vi "TestAndSetNextTestCasePointer.vi"(0 "TestSeqClass in":refnum<class "TestSeqClass.lvclass">, 11 "error in (no error)":errorcluster) -> (4 "TestSeqClass out":refnum<class "TestSeqClass.lvclass">, 8 "Continue":bool, 10 "Pointer at end":bool, 15 "error out":errorcluster)   [LabVIEW 2019, in "TestSeqClass.lvclass"]
uses:
  TestSeqClass.lvclass
  Typedef/TestStatus.ctl
  TestSeqClass.lvclass/TestSeqClass.ctl
  TestMeasureStep/TestMeasureStep.lvclass
  Read CurrentTestPointer.vi
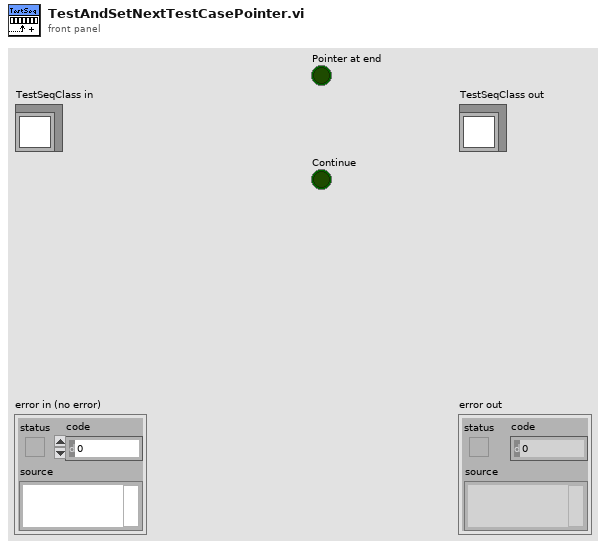
[diagram p1: front panel]
types:
  T1 = typedef "TestStatus.ctl" = enum16{"Not Executed", "Passed", "Failed", "Inconclusive", "Processing"}
  T2 = typedef "TestSeqType.ctl" = refnum<class "TestMeasureStep.lvclass">[]
  T3 = typedef "TestSeqClass.lvclass/TesstepType.ctl" = cluster{"TestName":string, "Meas":dbl, "Min ":dbl, "Max":dbl, "TestStatus":T1, "StringLimit":string, "StringMeas":string, "Unit":string}
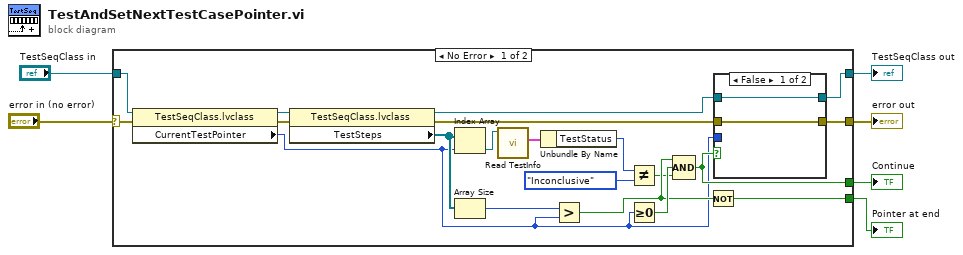
[diagram p0: block diagram]
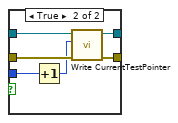
[diagram p2: hidden frame]
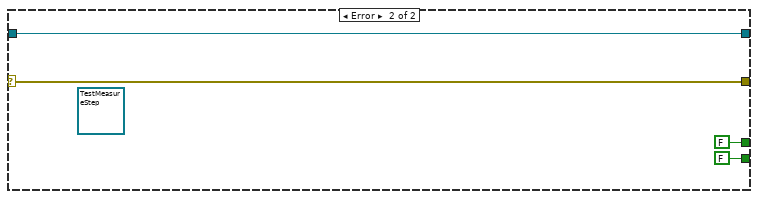
[diagram p3: hidden frame]
diagram:
  n1 = case shown="No Error" "error in (no error)" {
    selector: "error in (no error)" -> [w22 w38]
    tunnel: [w24 w38] -> w5
    tunnel: [w25 w37] -> w3
    tunnel: "TestSeqClass in" -> [w23 w37]
    tunnel: [w26 FALSE] -> w2
    tunnel: [w14 FALSE] -> w1
    frame No Error {
      n2 = property class="TestSeqClass.lvclass"(reference=w23, error in=w22) -> (reference out=w21:refnum<class "TestSeqClass.lvclass">, error out=w20:errorcluster, "CurrentTestPointer"=w12:u32)
      n3 = property class="TestSeqClass.lvclass"(reference=w21, error in=w20) -> (reference out=w17:refnum<class "TestSeqClass.lvclass">, error out=w16:errorcluster, "TestSteps"=w13:T2)
      n4 = Index Array(array=w13, index=w12) -> (element=w11:refnum<class "TestMeasureStep.lvclass">)
      n5 = Array Size(array=w13) -> (size(s)=w19:i32)
      n6 = call-dynamic "Read TestInfo.vi"("TestMeasureStep in"=w11) -> ("TestInfo 2"=w10:T3)  [unwired: 8 in, 2 out]
      n7 = Unbundle By Name(w10) -> ("TestStatus"=w9:T1)
      n8 = Greater?(x=w19, y=w12) -> (0:w15:bool)
      n9 = Not Equal?(x=w9, y=TestStatus."Inconclusive") -> (x != y?=w7:bool)
      n10 = Greater Or Equal To 0?(x=w12) -> (x >= 0?=w18:bool)
      n11 = Compound Arithmetic op=AND(w15, w18, w7) -> (w26:bool)
      n12 = Not(x=w15) -> (.not. x?=w14:bool)
      n13 = case shown="False" w26 {
        tunnel: w17 -> [w28 w34]
        tunnel: w16 -> [w27 w32]
        tunnel: w12 -> [_ w30]
        tunnel: [w28 w33] -> w25
        tunnel: [w27 w31] -> w24
        frame False {
        }
        frame True {
          n14 = Increment(x=w30) -> (x+1=w29:u32)
          n15 = call "Write CurrentTestPointer.vi"("error in (no error)"=w32, "CurrentTestPointer"=w29, "TestSeqClass in"=w34) -> ("error out"=w31:errorcluster, "TestSeqClass out"=w33:refnum<class "TestSeqClass.lvclass">)  [unwired: 7 in]
        }
      }
    }
    frame Error {
      (unwired) refnum<class "TestMeasureStep.lvclass"> refnum ("TestMeasureStep.lvclass")
    }
  }
  "error out" <- w5
  "TestSeqClass out" <- w3
  "Continue" <- w2
  "Pointer at end" <- w1
